vi "AI_wydobadz opisy.vi"(8 "error in (no error)":errorcluster, 10 "AI param aktywne in":T1[](array[typedef]) {"Numer" min=1 max=8 step=1}) -> (0 "error out":errorcluster, 1 "AI opisy out":string[](array[string]))   [LabVIEW 2013]
doc: "Wyciąga opisy\nz aktywnych kanałów analogowych"
uses:
  Kontrolki/GUI/AI_parametry.ctl
  Kontrolki/GUI/AI_wartosc.ctl
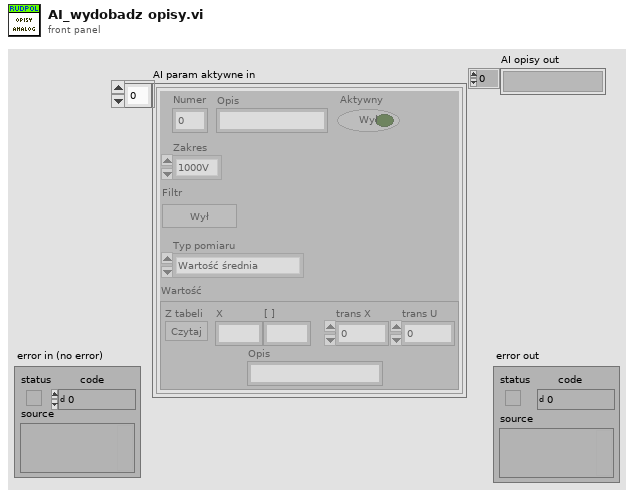
[diagram p1: front panel]
types:
  T1 = typedef "AI_parametry.ctl" = cluster{"Numer":u8, "Opis":string, "Zakres":enum16{"1000V", "300V", "30V", "3V", "0,3V"}, "Filtr":bool, "Typ pomiaru":enum16{"Wartość średnia", "Średnia wyprostowana", "Wartość skuteczna"}, "Aktywny":bool, "Wartość":T2}
  T2 = typedef "AI_wartosc.ctl" = cluster{"X":string, "[ ]":string, "trans X":dbl, "trans U":dbl, "Z tabeli":bool, "Opis":string}
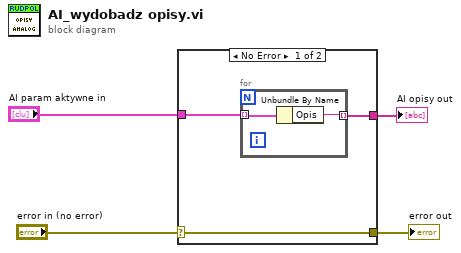
[diagram p0: block diagram]
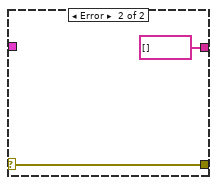
[diagram p2: hidden frame]
diagram:
  n1 = case shown="No Error" "error in (no error)" {
    selector: "error in (no error)" -> [w5 w11]
    tunnel: [w5 w11] -> w3
    tunnel: "AI param aktywne in" -> [w7 _]
    tunnel: [w6 string[] []] -> w1
    frame No Error {
      n2 = for {
        tunnel: w7 -> [w9] mode=indexing
        tunnel: [w8] -> w6 mode=indexing
        n3 = Unbundle By Name(w9) -> ("Opis"=w8:string)
      }
    }
    frame Error {
    }
  }
  "error out" <- w3
  "AI opisy out" <- w1
